vi "startAgent.vi"(6 "receiver":string, 8 "error in (no error)":errorcluster, 9 "sender":string, 10 "MobileAgent":refnum<class "MoAgSy_AgentBase.lvclass">) -> (0 "error out":errorcluster)   [LabVIEW 2009, in "MoAgSy_Base.lvlib" / "MoAgSy_Factory.lvclass"]
uses:
  MoAgSy_Factory.lvclass
  MoAgSy_AgentBase/MoAgSy_AgentBase.lvclass
  MoAgSy_Message/MoAgSy_Message.lvclass
  <vilib>/lvdsc/NI_DSC.lvlib
  HGF_BaseClasses/HGF_Factory/HGF_Factory.lvclass
  MoAgSy_Base.lvlib
panel:
  out "Agent started?":string
  out "Message":string
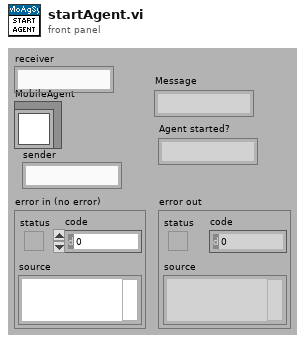
[diagram p1: front panel]
types:
  T1 = enum32{"u32BitField", "bool", "double", "string"}
  T2 = enum16{"key list", "pub key", "delete key", "add key", "local sign key"}
  T3 = enum16{"No Value", "Custom", "Double", "Boolean", "U32", "String", "DBL Array", "I32 Array", "I32", "SGL Array", "SGL", "I8", "U8", "I16", "U16", "I64", "U64", "DBL Waveform", "I16 Waveform", "Boolean Array", "I8 Array", "U8 Array", "I16 Array", "U16 Array", "U32 Array", "I64 Array", "U64 Array", "DBL Waveform Array", "I16 Waveform Array"}
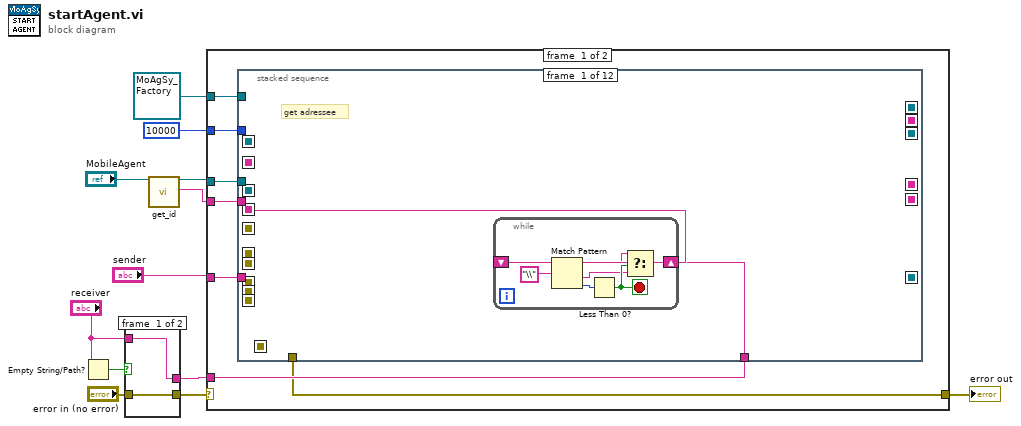
[diagram p0: block diagram]
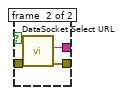
[diagram p2: hidden frame]
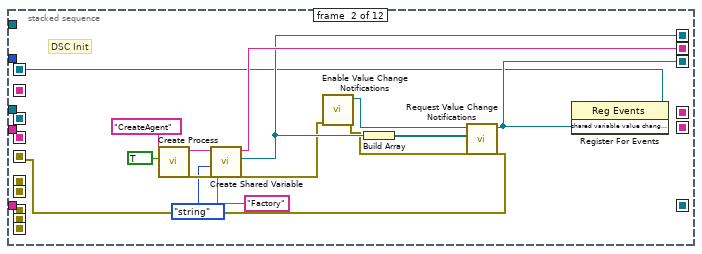
[diagram p3: hidden frame]
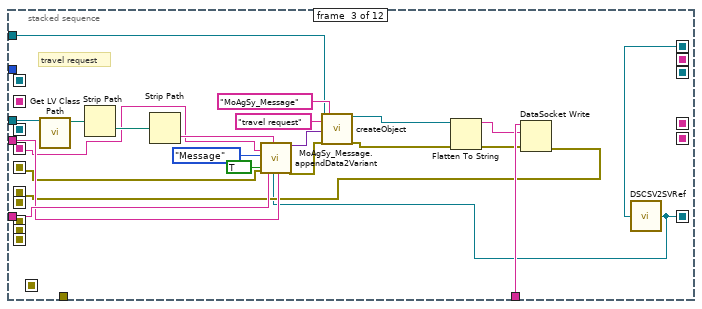
[diagram p4: hidden frame]
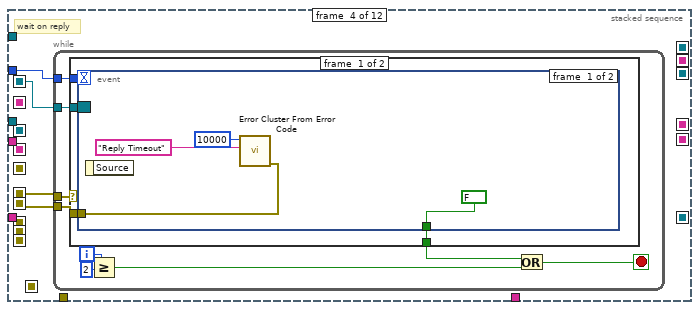
[diagram p5: hidden frame]
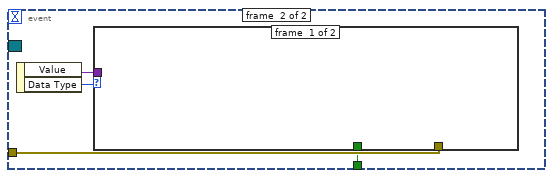
[diagram p6: hidden frame]
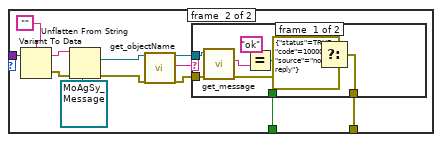
[diagram p7: hidden frame]
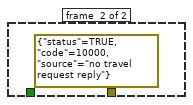
[diagram p8: hidden frame]
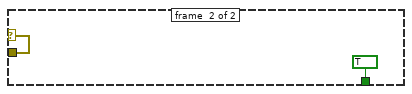
[diagram p9: hidden frame]
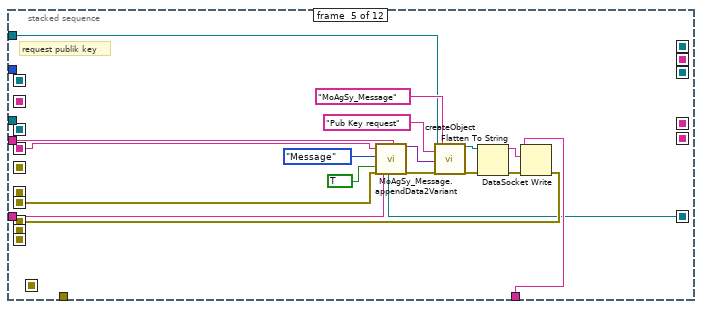
[diagram p10: hidden frame]
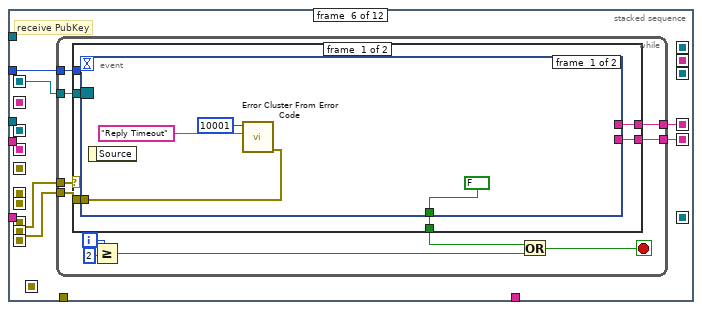
[diagram p11: hidden frame]
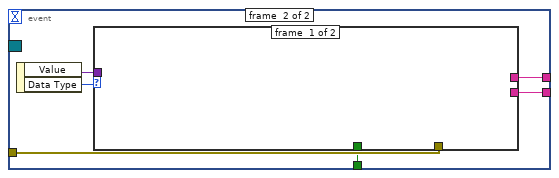
[diagram p12: hidden frame]
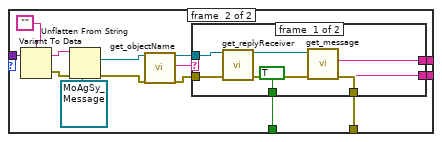
[diagram p13: hidden frame]
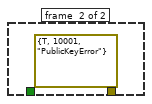
[diagram p14: hidden frame]
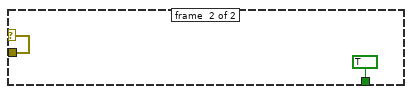
[diagram p15: hidden frame]
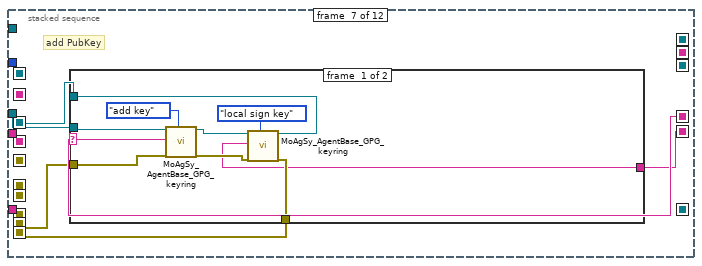
[diagram p16: hidden frame]
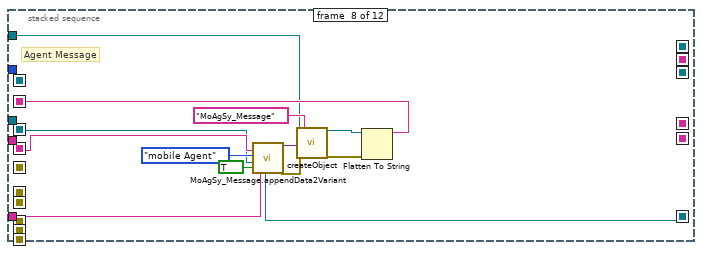
[diagram p18: hidden frame]
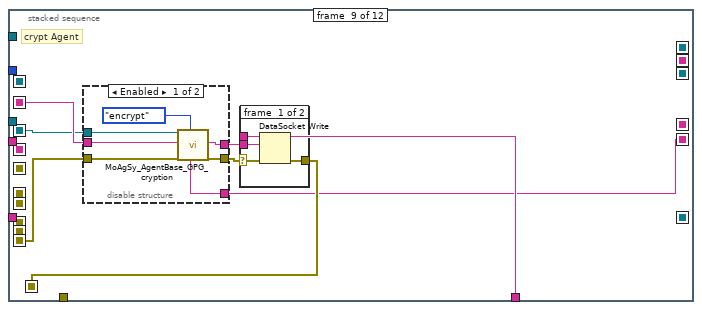
[diagram p19: hidden frame]
diagram:
  n1 = Empty String/Path?(string/path="receiver") -> (empty?=w3:bool)
  n2 = case shown="True" w3 {
    tunnel: [w13 w17] -> w11
    tunnel: "error in (no error)" -> [w14 w16]
    tunnel: [w14 w15] -> w9
    tunnel: "receiver" -> [w13 _]
    frame #0 {
    }
    frame #1 {
      n3 = call <vilib>:"DataSocket Select URL.vi"("error in (no error)"=w16) -> ("error out"=w15:errorcluster, "URL"=w17:string)  [unwired: 8 in, 1 out]
    }
  }
  n4 = call "get_id.vi"("HGF_Agent in"="MobileAgent") -> ("HGF_Agent out"=w7:refnum<class "MoAgSy_AgentBase.lvclass">, "ID"=w6:string)  [unwired: 16 in, 1 out]
  n5 = case shown="No Error" w9 {
    selector: w9 -> [_ w344]
    tunnel: [w19 w344] -> w12
    tunnel: w7 -> [w24 _]
    tunnel: w11 -> [w20 _]
    tunnel: w6 -> [w22 _]
    tunnel: "sender" -> [w23 _]
    tunnel: 10000 ("timeout") -> [w21 _]
    tunnel: refnum<class "MoAgSy_Factory.lvclass"> refnum ("MoAgSy_Factory in") -> [w18 _]
    frame #0 {
      n6 = stacked-sequence {
        seq-local: [_ w42 _ _ _ _ _ _ _ _ _ _] -> [_ _ _ _ _ _ _ _ _ _ _ w343]
        seq-local: [_ w41 _ _ _ _ _ _ _ _ _ _] -> [_ _ w51 _ _ _ _ _ _ _ _ w342]
        seq-local: [_ w34 _ _ _ _ _ _ _ _ _ _] -> [_ _ _ w73 _ w142 _ _ _ w248 w293 w338]
        seq-local: [_ w36 _ _ _ _ _ _ _ _ _ _] -> [_ _ w60 _ _ _ _ _ _ _ _ w337]
        seq-local: [_ _ w53 _ _ _ _ _ _ _ _ _] -> [_ _ _ w75 _ _ _ _ _ _ _ _]
        seq-local: [_ w35 _ _ _ _ _ _ _ _ _ _] -> [_ _ _ _ _ _ _ _ _ _ _ w339]
        seq-local: [_ _ _ w74 _ _ _ _ _ _ _ _] -> [_ _ _ _ w129 _ _ _ _ _ _ _]
        seq-local: [_ _ _ _ w123 _ _ _ _ _ _ _] -> [_ _ _ _ _ w140 _ _ _ _ _ _]
        seq-local: [_ _ _ _ _ w143 _ _ _ _ _ _] -> [_ _ _ _ _ _ w200 _ _ _ _ _]
        seq-local: [_ _ _ _ _ w139 _ _ _ _ _ _] -> [_ _ _ _ _ _ w198 _ _ _ _ _]
        seq-local: [_ _ _ _ _ _ w197 _ _ _ _ _] -> [_ _ _ _ _ _ _ _ w228 _ _ _]
        seq-local: [_ _ _ _ _ _ _ w216 _ _ _ _] -> [_ _ _ _ _ _ _ _ w232 _ _ _]
        seq-local: [_ _ _ _ _ _ _ _ w229 _ _ _] -> [_ _ _ _ _ _ _ _ _ w247 w292 _]
        seq-local: [w26 _ _ _ _ _ _ _ _ _ _ _] -> [_ _ w52 _ w122 _ _ w215 _ _ _ _]
        seq-local: [_ _ w50 _ _ _ _ _ _ _ _ _] -> [_ _ _ _ w121 _ _ w214 _ _ _ _]
        seq-local: [_ _ _ _ _ _ w196 _ _ _ _ _] -> [_ _ _ _ _ _ _ w213 w227 _ _ _]
        seq-local: [_ _ _ _ _ w138 _ _ _ _ _ _] -> [_ _ _ _ _ _ w195 _ w225 _ _ _]
        tunnel: w24 -> [_ _ w69 _ _ _ w199 _ _ _ _ _]
        tunnel: w23 -> [_ _ w62 _ w132 _ _ w220 _ _ _ _]
        tunnel: w22 -> [_ _ w61 _ w131 _ _ _ _ _ _ _]
        tunnel: w21 -> [_ _ _ w72 _ w141 _ _ _ w249 w294 _]
        tunnel: w20 -> [w25 _ w57 _ w124 _ _ _ w230 _ _ _]
        tunnel: [_ _ _ _ _ _ _ _ _ _ w291 _] -> w19
        tunnel: w18 -> [_ _ w49 _ w120 _ _ w212 _ _ _ _]
        frame #0 {
          # "get adressee"
          n7 = while {
            shift-right: [w27] -> w26
            shift-left: w25 -> [w33]
            stop <- w30 stop-if-true
            n8 = Match Pattern(string=w33, regular expression="\\") -> (before substring=w28:string, after substring=w29:string, offset past match=w32:i32)  [unwired: 1 in, 1 out]
            n9 = Less Than 0?(x=w32) -> (x < 0?=w30:bool)
            n10 = Select(t=w28, s=w30, f=w29) -> (s? t:f=w27:string)
          }
        }
        frame #1 {
          # "DSC Init"
          n11 = call <vilib>:"Create Process.vi"("run?"=TRUE, "process name"="CreateAgent") -> ("error out"=w44:errorcluster, "process name out"=w46:string)  [unwired: 8 in]
          n12 = call <vilib>:"Create Shared Variable.vi"("error in (no error)"=w44, "data type"=T1."string", "shared variable name"="Factory", "process name"=w46) -> ("error out"=w38:errorcluster, "shared variable"=w41:refnum<k21>, "process name out"=w42:string)  [unwired: 5 in]
          n13 = call <vilib>:"Enable Value Change Notifications.vi"("error in (no error)"=w38) -> ("error out"=w37:errorcluster, "shared variable value change notification"=w39:refnum<user-event>)  [unwired: 9 in]
          n14 = Build Array(w41) -> (w40:refnum<k21>[])
          n15 = call <vilib>:"Request Value Change Notifications.vi"("error in (no error)"=w37, "shared variables"=w40, "notification refnum"=w39) -> ("error out"=w36:errorcluster, "shared variable value change notification"=w35:refnum<user-event>)  [unwired: 6 in, 1 out]
          n16 = register-events(w35) -> (reference out=w34:refnum<event-registration>)  [unwired: 2 in, 1 out]
        }
        frame #2 {
          # "travel request"
          n17 = call <vilib>:"Get LV Class Path.vi"("object"=w69) -> ("class path"=w71:path)  [unwired: 1 in, 9 out]
          n18 = Strip Path(path=w71) -> (stripped path=w70:path)  [unwired: 1 out]
          n19 = Strip Path(path=w70) -> (name=w64:string)  [unwired: 1 out]
          n20 = call "DSCSV2SVRef.vi"("Shared Variable Control"=w51) -> ("shared variable refnum"=w50:refnum<k21>)
          n21 = call "MoAgSy_Message.appendData2Variant.vi"("addressee"=w52, "type"=enum16{"mobile Agent", "Visitor", "Message"}."Message", "request reply"=TRUE, "error in"=w60, "sender"=w62, "message"=w64, "reply to"=w50, "reply id"=w61) -> ("dup_initData"=w65:variant, "error out"=w59:errorcluster)  [unwired: 10 in]
          n22 = call "createObject.vi"("HGF_Factory"=w49, "objectName"="travel request", "initializationData"=w65, "error in (no error)"=w59, "className"="MoAgSy_Message") -> ("HGF_Object"=w58:refnum<class "HGF_Factory.lvclass">, "error out"=w54:errorcluster)  [unwired: 12 in, 1 out]
          n23 = Flatten To String(anything=w58, error in (no error)=w54) -> (data string=w56:string, error out=w55:errorcluster)  [unwired: 2 in, 1 out]
          n24 = DataSocket Write(8:w55, 10:w56, 11:w57) -> (0:w53:errorcluster)  [unwired: 1 in, 2 out]
        }
        frame #3 {
          # "wait on reply"
          n25 = while {
            tunnel: w75 -> [w84]
            tunnel: [w83] -> w74
            tunnel: w73 -> [w82]
            tunnel: w72 -> [w81]
            i -> [w78]
            stop <- w80 stop-if-true
            n26 = case shown="No Error" w84 {
              selector: w84 -> [_ w119]
              tunnel: [w86 w119] -> w83
              tunnel: w82 -> [w88 _]
              tunnel: w81 -> [w87 _]
              tunnel: [w85 TRUE] -> w79
              frame #0 {
                n27 = event shown="[1] <shared variable value change notification>: User Event" {
                  selector: w88 -> [_ _]
                  dyn-events: _ -> [_ _]
                  timeout: w87 -> [_ _]
                  tunnel: [w92 w95] -> w86
                  tunnel: [FALSE w93] -> w85
                  event #0 {
                    n28 = event-data() -> ()  [unwired: 1 in, 1 out]
                    n29 = call <vilib>:"Error Cluster From Error Code.vi"("error message (\"\")"="Reply Timeout" ("error message (\"\")"), "error code (0)"=10000) -> ("error out"=w92:errorcluster)  [unwired: 7 in]
                  }
                  event #1 {
                    n30 = event-data() -> ("Value"=w96:variant, "Data Type"=w94:T3)  [unwired: 1 in]
                    n31 = case shown="\"String\"" w94 {
                      tunnel: w96 -> [_ w108]
                      tunnel: [_ w103] -> w95
                      tunnel: [_ w98] -> w93
                      frame #0 {
                      }
                      frame #1 {
                        n32 = Variant To Data(Variant=w108, type="") -> (error out=w106:errorcluster, data=w105:string)  [unwired: 1 in]
                        n33 = Unflatten From String(type=refnum<class "MoAgSy_Message.lvclass"> refnum ("MoAgSy.lvlib:MoAgSy_Message.lvclass"), binary string=w105, error in (no error)=w106) -> (value=w100:refnum<class "MoAgSy_Message.lvclass">, error out=w102:errorcluster)  [unwired: 2 in, 1 out]
                        n34 = call "get_objectName.vi"("HGF_Factory"=w100, "error in (no error)"=w102) -> ("dup HGF_Factory"=w97:refnum<class "MoAgSy_Message.lvclass">, "objectName"=w99:string, "error out"=w101:errorcluster)  [unwired: 15 in]
                        n35 = case shown="\"reply\"" w99 {
                          tunnel: w101 -> [w115 _]
                          tunnel: [w110 errorcluster {"status"=TRUE, "code"=10000, "source"="no travel request reply"} ("error out")] -> w103
                          tunnel: [w112 _] -> w98
                          tunnel: w97 -> [w116 _]
                          frame #0 {
                            n36 = call "get_message.vi"("error in (no error)"=w115, "MoAgSy_Message.lvclass in"=w116) -> ("error out"=w111:errorcluster, "Message"=w114:string)  [unwired: 7 in, 1 out]
                            n37 = Equal?(x="ok" ("Message"), y=w114) -> (x = y?=w112:bool)
                            n38 = Select(t=w111, s=w112, f=errorcluster {"status"=TRUE, "code"=10000, "source"="no ok reply"}) -> (s? t:f=w110:errorcluster)
                          }
                          frame #1 {
                          }
                        }
                      }
                    }
                  }
                }
              }
              frame #1 {
              }
            }
            n39 = Greater Or Equal?(x=w78, y=2) -> (x >= y?=w76:bool)
            n40 = Or(x=w79, y=w76) -> (x .or. y?=w80:bool)
          }
        }
        frame #4 {
          # "request publik key"
          n41 = call "MoAgSy_Message.appendData2Variant.vi"("addressee"=w122, "type"=enum16{"mobile Agent", "Visitor", "Message"}."Message", "request reply"=TRUE, "error in"=w129, "sender"=w132, "reply to"=w121, "reply id"=w131) -> ("dup_initData"=w134:variant, "error out"=w130:errorcluster)  [unwired: 11 in]
          n42 = call "createObject.vi"("HGF_Factory"=w120, "objectName"="Pub Key request", "initializationData"=w134, "error in (no error)"=w130, "className"="MoAgSy_Message") -> ("HGF_Object"=w127:refnum<class "HGF_Factory.lvclass">, "error out"=w128:errorcluster)  [unwired: 12 in, 1 out]
          n43 = Flatten To String(anything=w127, error in (no error)=w128) -> (data string=w125:string, error out=w126:errorcluster)  [unwired: 2 in, 1 out]
          n44 = DataSocket Write(8:w126, 10:w125, 11:w124) -> (0:w123:errorcluster)  [unwired: 1 in, 2 out]
        }
        frame #5 {
          # "receive PubKey"
          n45 = while {
            tunnel: w140 -> [w154]
            tunnel: [w153] -> w139
            tunnel: w142 -> [w152]
            tunnel: w141 -> [w151]
            tunnel: [w145] -> w143
            tunnel: [w144] -> w138
            i -> [w148]
            stop <- w150 stop-if-true
            n46 = case shown="No Error" w154 {
              selector: w154 -> [_ w194]
              tunnel: [w158 w194] -> w153
              tunnel: w152 -> [w160 _]
              tunnel: w151 -> [w159 _]
              tunnel: [w157 TRUE] -> w149
              tunnel: [w156 _] -> w145
              tunnel: [w155 _] -> w144
              frame #0 {
                n47 = event shown="[1] <shared variable value change notification>: User Event" {
                  selector: w160 -> [_ _]
                  dyn-events: _ -> [_ _]
                  timeout: w159 -> [_ _]
                  tunnel: [w164 w169] -> w158
                  tunnel: [FALSE w167] -> w157
                  tunnel: [_ w166] -> w156
                  tunnel: [_ w165] -> w155
                  event #0 {
                    n48 = event-data() -> ()  [unwired: 1 in, 1 out]
                    n49 = call <vilib>:"Error Cluster From Error Code.vi"("error message (\"\")"="Reply Timeout" ("error message (\"\")"), "error code (0)"=10001) -> ("error out"=w164:errorcluster)  [unwired: 7 in]
                  }
                  event #1 {
                    n50 = event-data() -> ("Value"=w170:variant, "Data Type"=w168:T3)  [unwired: 1 in]
                    n51 = case shown="\"String\"" w168 {
                      tunnel: w170 -> [_ w184]
                      tunnel: [_ w179] -> w169
                      tunnel: [_ w174] -> w167
                      tunnel: [_ w172] -> w166
                      tunnel: [_ w171] -> w165
                      frame #0 {
                      }
                      frame #1 {
                        n52 = Variant To Data(Variant=w184, type="") -> (error out=w182:errorcluster, data=w181:string)  [unwired: 1 in]
                        n53 = Unflatten From String(type=refnum<class "MoAgSy_Message.lvclass"> refnum ("MoAgSy.lvlib:MoAgSy_Message.lvclass"), binary string=w181, error in (no error)=w182) -> (value=w176:refnum<class "MoAgSy_Message.lvclass">, error out=w178:errorcluster)  [unwired: 2 in, 1 out]
                        n54 = call "get_objectName.vi"("HGF_Factory"=w176, "error in (no error)"=w178) -> ("dup HGF_Factory"=w173:refnum<class "MoAgSy_Message.lvclass">, "objectName"=w175:string, "error out"=w177:errorcluster)  [unwired: 15 in]
                        n55 = case shown="\"PublicKey\"" w175 {
                          tunnel: w177 -> [w191 _]
                          tunnel: [w189 errorcluster {"status"=TRUE, "code"=10001, "source"="PublicKeyError"} ("error out")] -> w179
                          tunnel: [TRUE _] -> w174
                          tunnel: w173 -> [w187 _]
                          tunnel: [w190 _] -> w172
                          tunnel: [w185 _] -> w171
                          frame #0 {
                            n56 = call "get_replyReceiver.vi"("MoAgSy_Message"=w187) -> ("sender ID"=w185:string, "dup MoAgSy_Message"=w186:refnum<class "MoAgSy_Message.lvclass">)  [unwired: 13 in, 4 out]
                            n57 = call "get_message.vi"("error in (no error)"=w191, "MoAgSy_Message.lvclass in"=w186) -> ("error out"=w189:errorcluster, "Message"=w190:string)  [unwired: 7 in, 1 out]
                          }
                          frame #1 {
                          }
                        }
                      }
                    }
                  }
                }
              }
              frame #1 {
              }
            }
            n58 = Greater Or Equal?(x=w148, y=2) -> (x >= y?=w146:bool)
            n59 = Or(x=w149, y=w146) -> (x .or. y?=w150:bool)
          }
        }
        frame #6 {
          # "add PubKey"
          n60 = case shown="Default" w200 {
            selector: w200 -> [w206 _]
            tunnel: w199 -> [w210 _]
            tunnel: w198 -> [w204 w211]
            tunnel: [w203 w211] -> w197
            tunnel: [w202 _] -> w196
            tunnel: w195 -> [w201 _]
            frame #0 {
              n61 = call "MoAgSy_AgentBase_GPG_keyring.vi"("HGF_Agent in"=w210, "key"=w206, "error in (no error)"=w204, "Enum"=T2."add key") -> ("HGF_Agent out"=w207:refnum<class "MoAgSy_AgentBase.lvclass">, "error out"=w208:errorcluster)  [unwired: 12 in, 2 out]
              n62 = call "MoAgSy_AgentBase_GPG_keyring.vi"("HGF_Agent in"=w207, "key"=w201, "error in (no error)"=w208, "Enum"=T2."local sign key") -> ("HGF_Agent out"=w202:refnum<class "MoAgSy_AgentBase.lvclass">, "error out"=w203:errorcluster)  [unwired: 12 in, 2 out]
            }
            frame #1 {
            }
          }
        }
        frame #7 {
          # "Agent Message"
          n63 = call "MoAgSy_Message.appendData2Variant.vi"("addressee"=w215, "type"=enum16{"mobile Agent", "Visitor", "Message"}."mobile Agent", "Object"=w213, "request reply"=TRUE, "sender"=w220, "reply to"=w214) -> ("dup_initData"=w222:variant, "error out"=w219:errorcluster)  [unwired: 12 in]
          n64 = call "createObject.vi"("HGF_Factory"=w212, "initializationData"=w222, "error in (no error)"=w219, "className"="MoAgSy_Message") -> ("HGF_Object"=w217:refnum<class "HGF_Factory.lvclass">, "error out"=w218:errorcluster)  [unwired: 13 in, 1 out]
          n65 = Flatten To String(anything=w217, error in (no error)=w218) -> (data string=w216:string)  [unwired: 2 in, 2 out]
        }
        frame #8 {
          # "crypt Agent"
          n66 = disable-structure shown="Enabled" {
            disable-tunnel: w232 -> [w239 w241]
            disable-tunnel: [w237 w241] -> w231
            disable-tunnel: w228 -> [w236 w240]
            disable-tunnel: w227 -> [w235 _]
            disable-tunnel: [w234 w240] -> w226
            disable-tunnel: w225 -> [w233 _]
            frame #0 {
              n67 = call "MoAgSy_AgentBase_GPG_cryption.vi"("HGF_Agent in"=w235, "string in"=w239, "error in (no error)"=w236, "task"=enum16{"encrypt", "decrypt", "sign", "verify"}."encrypt", "receiver"=w233) -> ("String out"=w237:string, "error out"=w234:errorcluster)  [unwired: 11 in, 2 out]
            }
            frame #1 {
            }
          }
          n68 = case shown="No Error" w226 {
            selector: w226 -> [w242 w246]
            tunnel: w231 -> [w244 _]
            tunnel: w230 -> [w245 _]
            tunnel: [w243 w246] -> w229
            frame #0 {
              n69 = DataSocket Write(8:w242, 10:w244, 11:w245) -> (0:w243:errorcluster)  [unwired: 1 in, 2 out]
            }
            frame #1 {
            }
          }
        }
        frame #9 {
          # "receive host reply"
          n70 = while {
            tunnel: [w258] -> _
            tunnel: w249 -> [w252]
            tunnel: w248 -> [w251]
            tunnel: w247 -> [w250]
            i -> [w255]
            stop <- w257 stop-if-true
            n71 = case shown="No Error" w250 {
              selector: w250 -> [_ w290]
              tunnel: [w262 w290] -> w258
              tunnel: [w261 TRUE] -> w256
              tunnel: w252 -> [w260 _]
              tunnel: w251 -> [w259 _]
              frame #0 {
                n72 = event shown="[1] <shared variable value change notification>: User Event" {
                  selector: w259 -> [_ _]
                  dyn-events: _ -> [_ _]
                  timeout: w260 -> [_ _]
                  tunnel: [w266 w269] -> w262
                  tunnel: [FALSE w267] -> w261
                  event #0 {
                    n73 = event-data() -> ()  [unwired: 1 in, 1 out]
                    n74 = call <vilib>:"Error Cluster From Error Code.vi"("error message (\"\")"="Reply Timeout" ("error message (\"\")"), "error code (0)"=10000) -> ("error out"=w266:errorcluster)  [unwired: 7 in]
                  }
                  event #1 {
                    n75 = event-data() -> ("Value"=w270:variant, "Data Type"=w268:T3)  [unwired: 1 in]
                    n76 = case shown="\"String\"" w268 {
                      tunnel: w270 -> [_ w282]
                      tunnel: [_ w277] -> w269
                      tunnel: [_ w272] -> w267
                      frame #0 {
                      }
                      frame #1 {
                        n77 = Variant To Data(Variant=w282, type="") -> (error out=w280:errorcluster, data=w279:string)  [unwired: 1 in]
                        n78 = Unflatten From String(type=refnum<class "MoAgSy_Message.lvclass"> refnum ("MoAgSy.lvlib:MoAgSy_Message.lvclass"), binary string=w279, error in (no error)=w280) -> (value=w274:refnum<class "MoAgSy_Message.lvclass">, error out=w276:errorcluster)  [unwired: 2 in, 1 out]
                        n79 = call "get_objectName.vi"("HGF_Factory"=w274, "error in (no error)"=w276) -> ("dup HGF_Factory"=w271:refnum<class "MoAgSy_Message.lvclass">, "objectName"=w273:string, "error out"=w275:errorcluster)  [unwired: 15 in]
                        n80 = case shown="\"reply\"" w273 {
                          tunnel: w275 -> [w286 _]
                          tunnel: [w285 errorcluster {"status"=TRUE, "code"=10002, "source"="no received reply"} ("error out")] -> w277
                          tunnel: [TRUE _] -> w272
                          tunnel: w271 -> [w287 _]
                          frame #0 {
                            n81 = call "get_message.vi"("error in (no error)"=w286, "MoAgSy_Message.lvclass in"=w287) -> ("error out"=w285:errorcluster, "Message"=→"Message":string)  [unwired: 7 in, 1 out]
                          }
                          frame #1 {
                          }
                        }
                      }
                    }
                  }
                }
              }
              frame #1 {
              }
            }
            n82 = Greater Or Equal?(x=w255, y=2) -> (x >= y?=w253:bool)
            n83 = Or(x=w256, y=w253) -> (x .or. y?=w257:bool)
          }
        }
        frame #10 {
          # "receive start agent message"
          n84 = while {
            tunnel: [w303] -> w291
            tunnel: w294 -> [w297]
            tunnel: w293 -> [w296]
            tunnel: w292 -> [w295]
            i -> [w300]
            stop <- w302 stop-if-true
            n85 = case shown="No Error" w295 {
              selector: w295 -> [_ w335]
              tunnel: [w307 w335] -> w303
              tunnel: [w306 TRUE] -> w301
              tunnel: w297 -> [w305 _]
              tunnel: w296 -> [w304 _]
              frame #0 {
                n86 = event shown="[1] <shared variable value change notification>: User Event" {
                  selector: w304 -> [_ _]
                  dyn-events: _ -> [_ _]
                  timeout: w305 -> [_ _]
                  tunnel: [w311 w314] -> w307
                  tunnel: [FALSE w312] -> w306
                  event #0 {
                    n87 = event-data() -> ()  [unwired: 1 in, 1 out]
                    n88 = call <vilib>:"Error Cluster From Error Code.vi"("error message (\"\")"="Reply Timeout" ("error message (\"\")"), "error code (0)"=10000) -> ("error out"=w311:errorcluster)  [unwired: 7 in]
                  }
                  event #1 {
                    n89 = event-data() -> ("Value"=w315:variant, "Data Type"=w313:T3)  [unwired: 1 in]
                    n90 = case shown="\"String\"" w313 {
                      tunnel: w315 -> [_ w327]
                      tunnel: [_ w322] -> w314
                      tunnel: [_ w317] -> w312
                      frame #0 {
                      }
                      frame #1 {
                        n91 = Variant To Data(Variant=w327, type="") -> (error out=w325:errorcluster, data=w324:string)  [unwired: 1 in]
                        n92 = Unflatten From String(type=refnum<class "MoAgSy_Message.lvclass"> refnum ("MoAgSy.lvlib:MoAgSy_Message.lvclass"), binary string=w324, error in (no error)=w325) -> (value=w319:refnum<class "MoAgSy_Message.lvclass">, error out=w321:errorcluster)  [unwired: 2 in, 1 out]
                        n93 = call "get_objectName.vi"("HGF_Factory"=w319, "error in (no error)"=w321) -> ("dup HGF_Factory"=w316:refnum<class "MoAgSy_Message.lvclass">, "objectName"=w318:string, "error out"=w320:errorcluster)  [unwired: 15 in]
                        n94 = case shown="\"reply\"" w318 {
                          tunnel: w320 -> [w331 _]
                          tunnel: [w330 errorcluster {"status"=TRUE, "code"=10002, "source"="no received reply"} ("error out")] -> w322
                          tunnel: [TRUE _] -> w317
                          tunnel: w316 -> [w332 _]
                          frame #0 {
                            n95 = call "get_message.vi"("error in (no error)"=w331, "MoAgSy_Message.lvclass in"=w332) -> ("error out"=w330:errorcluster, "Message"=→"Agent started?":string)  [unwired: 7 in, 1 out]
                          }
                          frame #1 {
                          }
                        }
                      }
                    }
                  }
                }
              }
              frame #1 {
              }
            }
            n96 = Greater Or Equal?(x=w300, y=2) -> (x >= y?=w298:bool)
            n97 = Or(x=w301, y=w298) -> (x .or. y?=w302:bool)
          }
        }
        frame #11 {
          # "DSC DeInit"
          n98 = Unregister For Events(event registration refnum=w338, error in=w337) -> (error out=w336:errorcluster)
          n99 = call <vilib>:"Disable Value Change Notifications.vi"("error in (no error)"=w336, "notification refnum"=w339) -> ("error out"=w341:errorcluster)  [unwired: 9 in]
          n100 = call <vilib>:"Delete Shared Variable.vi"("error in (no error)"=w341, "shared variable"=w342) -> ("error out"=w340:errorcluster)  [unwired: 9 in]
          n101 = call <vilib>:"Delete Process.vi"("error in (no error)"=w340, "process name"=w343) -> ()  [unwired: 9 in, 1 out]
        }
      }
    }
    frame #1 {
    }
  }
  "error out" <- w12
